vi "Characteristic.vi"(5 "EndTime":timestamp, 7 "StartTime":timestamp, 8 "error in (no error)":errorcluster, 11 "Characteristic in":refnum<class "Characteristic.lvclass">) -> (0 "error out":errorcluster, 3 "Passed":bool)   [LabVIEW 2020]
uses:
  ProligentResultProcessor/Model/Characteristic/Characteristic.lvclass
  ProligentResultProcessor/Model/Characteristic/SetFullName.vi
  ProligentResultProcessor/Model/Characteristic/SetValue.vi
  ProligentResultProcessor/Model/Characteristic/GetFullName.vi
  ProligentResultProcessor/Model/Characteristic/GetValue.vi
  ProligentResultProcessor/Model/Characteristic/GetCustomData.vi
  ProligentResultProcessor/Model/CustomData/CustomData.lvclass
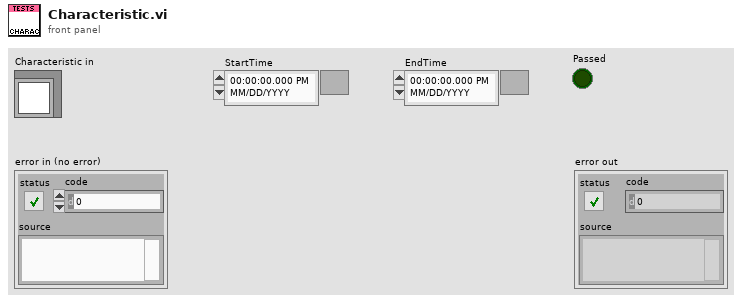
[diagram p1: front panel]
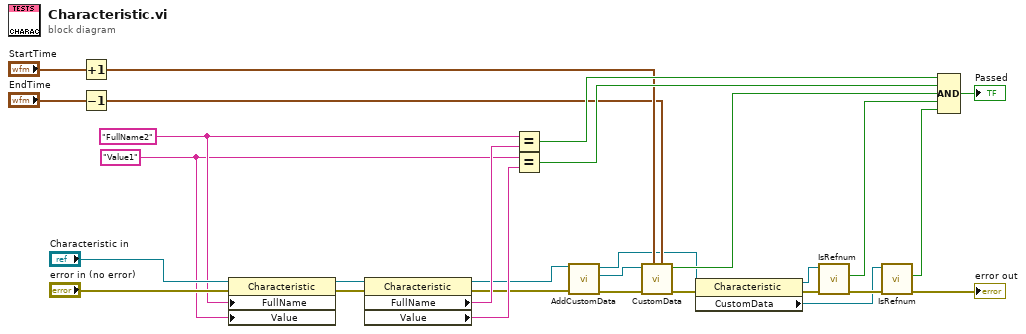
[diagram p0: block diagram]
diagram:
  w22 = "Value1"
  w24 = "FullName2"
  n1 = Increment(x="StartTime") -> (x+1=w13:timestamp)
  n2 = Decrement(x="EndTime") -> (x-1=w12:timestamp)
  n3 = property class="Characteristic"(reference="Characteristic in", error in="error in (no error)", "FullName"=w24, "Value"=w22) -> (reference out=w27:refnum<class "Characteristic.lvclass">, error out=w26:errorcluster)
  n4 = property class="Characteristic"(reference=w27, error in=w26) -> (reference out=w20:refnum<class "Characteristic.lvclass">, error out=w21:errorcluster, "FullName"=w25:string, "Value"=w23:string)
  n5 = Equal?(x=w24, y=w25) -> (x = y?=w19:bool)
  n6 = Equal?(x=w22, y=w23) -> (x = y?=w18:bool)
  n7 = call "AddCustomData.vi"("error in"=w21, "Document in"=w20) -> ("error out"=w16:errorcluster, "CustomData"=w17:refnum<class "CustomData.lvclass">, "Document out"=w7:refnum<class "Characteristic.lvclass">)  [unwired: 7 in]
  n8 = call "CustomData.vi"("EndTime"=w12, "StartTime"=w13, "error in"=w16, "CustomData"=w17) -> ("error out"=w10:errorcluster, "Passed"=w11:bool)  [unwired: 6 in]
  n9 = property class="Characteristic"(reference=w7, error in=w10) -> (reference out=w6:refnum<class "Characteristic.lvclass">, error out=w8:errorcluster, "CustomData"=w3:refnum<class "CustomData.lvclass">)
  n10 = call "IsRefnum.vi"("error in"=w8, "Document in"=w6) -> ("error out"=w4:errorcluster, "IsRefnum"=w9:bool)  [unwired: 7 in, 1 out]
  n11 = call "IsRefnum.vi"("error in"=w4, "CustomDataType in"=w3) -> ("error out"=→"error out":errorcluster, "IsRefnum"=w2:bool)  [unwired: 7 in, 1 out]
  n12 = Compound Arithmetic op=AND(w19, w18, w11, w9, w2) -> (→"Passed":bool)
